vi "HapticSPM_read - Test Bench.vi"() -> ()   [LabVIEW 2019]
uses:
  <userlib>/HapticSTM/HapticSTM.lvlib
panel:
  in  "Fine Adjust":dbl(slide)=3.163265306122449 scale=0.0..10.0
  out "Value":sgl format="%.1p"
  in  "Index":i8
  out "Size (m)":cluster{"Width":sgl, "Height":sgl} {"Height" format="%.2p"; "Width" format="%.2p"}
  out "Origin (m)":cluster{"Xc":sgl, "Yc":sgl} {"Yc" format="%.2p"; "Xc" format="%.2p"}
  out "Positions":T1 {"z (mm)" format="%.1p"; "y (nm)" format="%.1p"; "x (nm)" format="%.1p"}
  out "Forces":T2 {"Fz (N)" format="%.1p"; "Fy (N)" format="%.1p"; "Fx (N)" format="%.1p"}
  in  "Save":bool
  out "Arm Output:":dbl format="%^.1g"
  in  "Rough Adjust":dbl
  in  "Drag":dbl=1.0
  in  "STOP":bool
  out "Clicks":dbl
  # "Read Mode - Haptic SPM"
  # "Signal"
  # "Sensitivity"
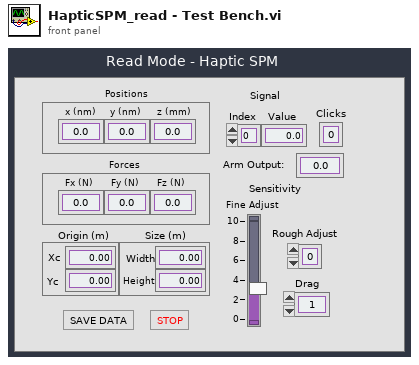
[diagram p1: front panel]
types:
  T1 = cluster{"x (nm)":dbl, "y (nm)":dbl, "z (mm)":dbl}
  T2 = cluster{"Fx (N)":dbl, "Fy (N)":dbl, "Fz (N)":dbl}
  T3 = cluster{"Xc":dbl, "Yc":dbl, "Width":dbl, "Height":dbl}
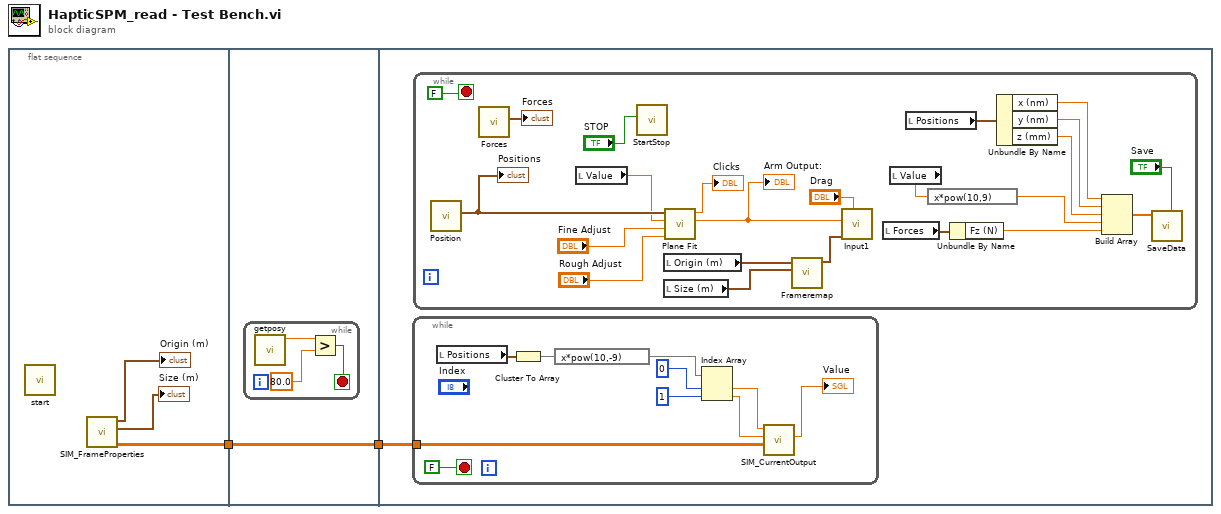
[diagram p0: block diagram]
diagram:
  n1 = flat-sequence {
    tunnel: [w3] -> w2
    tunnel: w2 -> [w6]
    tunnel: [w6] -> w1
    tunnel: w1 -> [w10]
    frame #0 {
      n2 = call <userlib>:"start.vi"() -> ()  [unwired: 11 in, 1 out]
      n3 = call "SIM_FrameProperties.vi"() -> ("data"=w3:dbl[][], "Size (m)"=→"Size (m)":cluster{"Width":sgl, "Height":sgl}, "Origin (m)"=→"Origin (m)":cluster{"Xc":sgl, "Yc":sgl})  [unwired: 9 in]
    }
    frame #1 {
      n4 = while {
        stop <- w7 stop-if-true
        n5 = call <userlib>:"getposy.vi"() -> ("function return"=w9:dbl)  [unwired: 11 in]
        n6 = Greater?(x=w9, y=80.0) -> (0:w7:bool)
      }
    }
    frame #2 {
      n7 = while {
        tunnel: w10 -> [w14]
        stop <- FALSE stop-if-true
        n8 = local read "Positions"() -> (w19:T1)
        n9 = Cluster To Array(cluster=w19) -> (array=w18:dbl[])
        n10 = expression code="x*pow(10,-9)"(w18) -> (w17:dbl[])
        n11 = Index Array(array=w17, index #1=0 ("index"), index #2=1 ("index")) -> (element #1=w12:dbl, element #2=w11:dbl)
        n12 = call "SIM_CurrentOutput.vi"("array"=w14, "y"=w11, "x"=w12) -> ("Zread"=→"Value":dbl)  [unwired: 8 in]
      }
      n13 = while {
        stop <- FALSE stop-if-true
        n14 = call "Position.vi"() -> ("Positions"=w39:T1)  [unwired: 11 in]
        "Positions" <- w39
        n15 = call "Forces.vi"() -> ("Forces"=→"Forces":T2)  [unwired: 11 in]
        n16 = local read "Value"() -> (w37:sgl)
        n17 = call "StartStop.vi"("STOP"="STOP") -> ()  [unwired: 11 in]
        n18 = local read "Origin (m)"() -> (w36:cluster{"Xc":sgl, "Yc":sgl})
        n19 = local read "Size (m)"() -> (w35:cluster{"Width":sgl, "Height":sgl})
        n20 = call "Plane Fit.vi"("Rough Adjust"="Rough Adjust", "Fine Adjust"="Fine Adjust", "Nano Z"=w37, "Positions"=w39) -> ("Output"=w24:dbl, "Clicks"=→"Clicks":dbl)  [unwired: 6 in]
        "Arm Output:" <- w24
        n21 = call "Frameremap.vi"("Size (m)"=w35, "Origin (m)"=w36) -> ("Remapped Frame Properties"=w23:T3)  [unwired: 9 in]
        n22 = call "Input1.vi"("Drag"="Drag", "Remapped Frame Properties"=w23, "Signal in"=w24) -> ()  [unwired: 9 in]
        n23 = local read "Forces"() -> (w27:T2)
        n24 = local read "Value"() -> (w29:sgl)
        n25 = local read "Positions"() -> (w33:T1)
        n26 = expression code="x*pow(10,9)"(w29) -> (w28:sgl)
        n27 = Unbundle By Name(w27) -> ("Fz (N)"=w26:dbl)
        n28 = Unbundle By Name(w33) -> ("x (nm)"=w32:dbl, "y (nm)"=w31:dbl, "z (mm)"=w30:dbl)
        n29 = Build Array(w32, w31, w30, w28, w26) -> (w25:dbl[])
        n30 = call "SaveData.vi"("Save"="Save", "Data"=w25) -> ()  [unwired: 10 in]
      }
    }
  }
